vi "get_xwav_attribute_by_name.vi"(8 "Error in":errorcluster caption="Error in (no error)", 10 "name":string, 11 "xwave in":T1={"attributes"=variant, "X"={"start"=0.0, "delta"=0.0, "units"="index", "dim"="au"}, "Y"={"data"=[], "units"="au"}}) -> (0 "Error out":errorcluster, 1 "value":variant, 2 "found?":bool, 3 "xwave out":T1={"attributes"=variant, "X"={"start"=0.0, "delta"=0.0, "units"="index", "dim"="au"}, "Y"={"data"=[], "units"="au"}})   [LabVIEW 2015]
uses:
  xwav.ctl
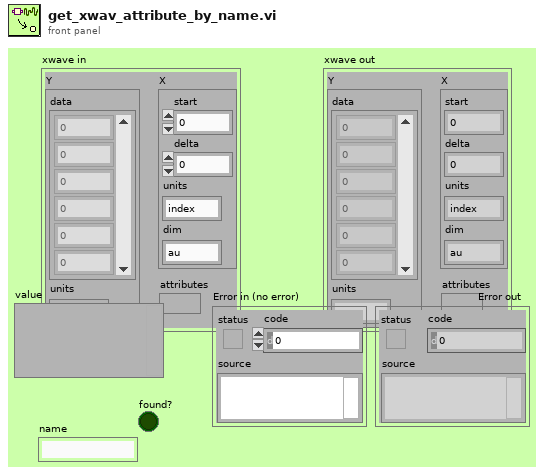
[diagram p1: front panel]
types:
  T1 = typedef "xwav.ctl" = cluster{"attributes":variant, "X":cluster{"start":dbl, "delta":dbl, "units":string, "dim":string}, "Y":cluster{"data":dbl[], "units":string}}
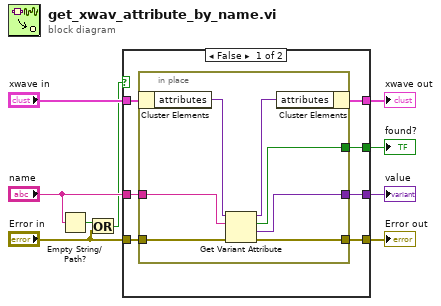
[diagram p0: block diagram]
diagram:
  n1 = Empty String/Path?(string/path="name") -> (empty?=w4:bool)
  n2 = Or(x=w4, y="Error in") -> (x .or. y?=w3:bool)
  n3 = case shown="False" w3 {
    tunnel: "xwave in" -> [w16 w25]
    tunnel: [w15 w25] -> w8
    tunnel: "name" -> [w14 _]
    tunnel: [w13 _] -> w6
    tunnel: [w12 _] -> w5
    tunnel: [w11 w24] -> w2
    tunnel: "Error in" -> [w10 w24]
    frame False {
      n4 = in-place {
        in-place-border: w14 -> [w21]
        in-place-border: [w20] -> w13
        in-place-border: [w19] -> w12
        in-place-border: [w18] -> w11
        in-place-border: w10 -> [w17]
        n5 = in-place-cluster #1(w16) -> ("attributes"=w23:variant)
        n6 = Get Variant Attribute(Variant=w23, name=w21, error in=w17) -> (duplicate Variant=w22:variant, found=w19:bool, value=w20:variant, error out=w18:errorcluster)  [unwired: 1 in]
        n7 = in-place-cluster #1("attributes"=w22) -> (w15:T1)
      }
    }
    frame True {
    }
  }
  "xwave out" <- w8
  "value" <- w6
  "found?" <- w5
  "Error out" <- w2
